vi "trainConGan.vi"(0 "error in (no error)":errorcluster, 1 "ptr_D":i64, 3 "ptr_G":i64, 4 "eta_D":sgl, 5 "eta_G":sgl, 7 "batch_update":u32, 8 "rmsProp":bool=TRUE, 9 "gamma":sgl, 10 "X":sgl[][](array[numeric]), 11 "Y":sgl[][](array[numeric]), 12 "adam":bool=TRUE, 13 "lambda":sgl, 14 "spectral norm discriminator":bool=TRUE, 15 "first Layer":u32, 16 "weight norm Generator":bool=TRUE, 17 "last layer":u32, 18 "train Gen":bool=TRUE, 19 "Gen to sidechannel":bool=TRUE, 27 "handOverLayer":u32) -> (20 "error out":errorcluster, 21 "ptr_D out":i64, 23 "ptr_G out":i64, 24 "Generator output":sgl[][](array[numeric]), 25 "D_REAL_ERR":sgl, 26 "D_FAKE_ERR":sgl)   [LabVIEW 2016, in "CNet.lvlib"]
uses:
  CNet.lvlib
  Users/jg754/Documents/Visual Studio 2015/Projects/CLearn/x64/Release/CLearn.dll
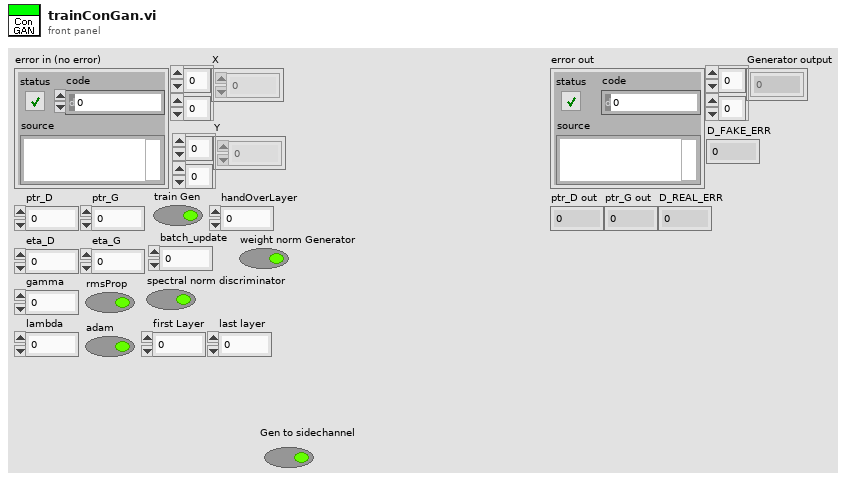
[diagram p1: front panel]
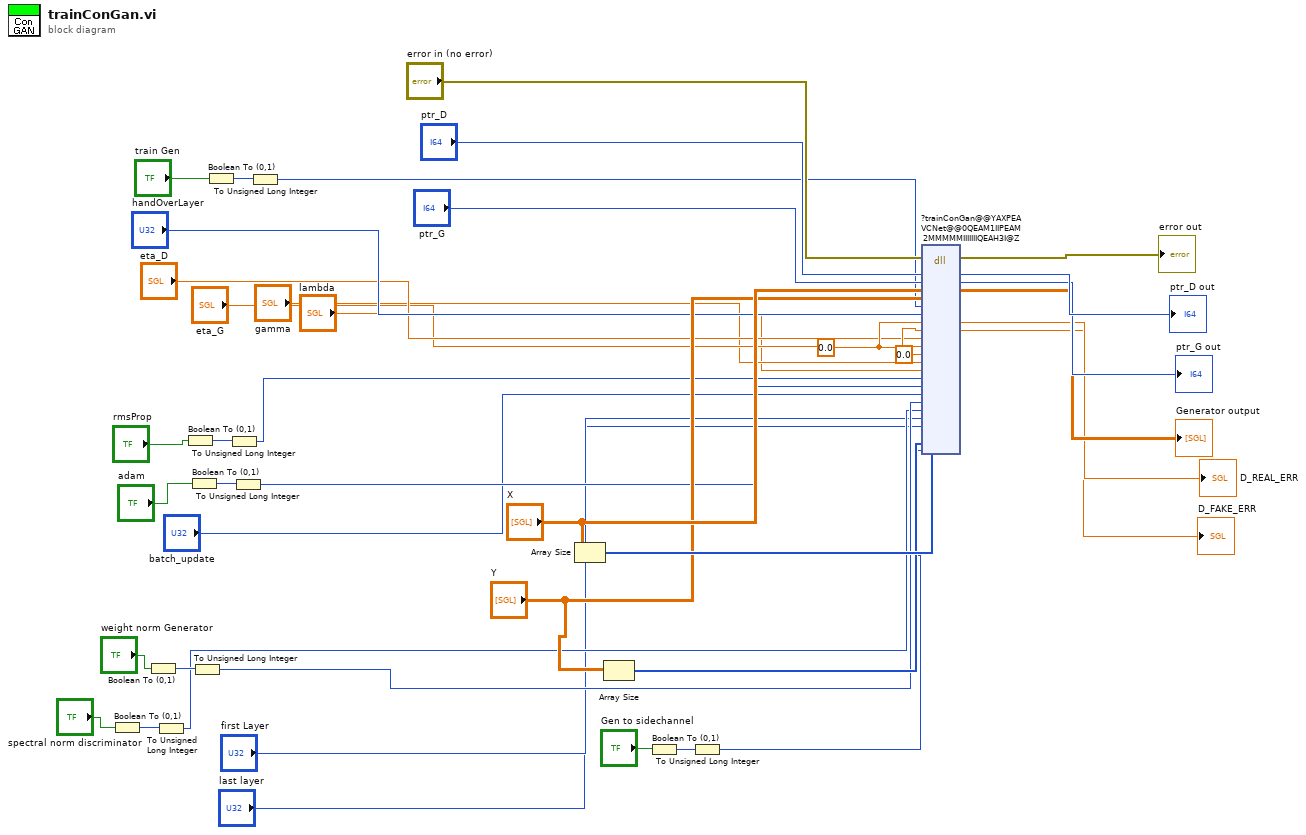
[diagram p0: block diagram]
diagram:
  w26 = sgl 0.0 ("D_REAL_ERR")
  n1 = Boolean To (0,1)(Boolean="spectral norm discriminator") -> (0, 1=w10:i16)
  n2 = Boolean To (0,1)(Boolean="weight norm Generator") -> (0, 1=w13:i16)
  n3 = To Unsigned Long Integer(number=w10) -> (unsigned 32bit integer=w8:u32)
  n4 = Boolean To (0,1)(Boolean="rmsProp") -> (0, 1=w20:i16)
  n5 = Boolean To (0,1)(Boolean="adam") -> (0, 1=w17:i16)
  n6 = To Unsigned Long Integer(number=w13) -> (unsigned 32bit integer=w11:u32)
  n7 = Boolean To (0,1)(Boolean="train Gen") -> (0, 1=w29:i16)
  n8 = To Unsigned Long Integer(number=w20) -> (unsigned 32bit integer=w18:u32)
  n9 = To Unsigned Long Integer(number=w17) -> (unsigned 32bit integer=w15:u32)
  n10 = To Unsigned Long Integer(number=w29) -> (unsigned 32bit integer=w28:u32)
  n11 = Array Size(array="X") -> (size(s)=w34:i32[])
  n12 = Array Size(array="Y") -> (size(s)=w32:i32[])
  n13 = Boolean To (0,1)(Boolean="Gen to sidechannel") -> (0, 1=w2:i16)
  n14 = To Unsigned Long Integer(number=w2) -> (unsigned 32bit integer=w1:u32)
  n15 = dll-call lib="C:/Users/jg754/Documents/Visual Studio 2015/Projects/CLearn/x64/Release/CLearn.dll" fn="?trainConGan@@YAXPEAVCNet@@0QEAM1IIPEAM2MMMMMIIIIIIIQEAH3I@Z"(error in="error in (no error)", "ptr_D"="ptr_D", "ptr_G"="ptr_G", "X"="X", "Y"="Y", "prepGen"=w28, "handOverLayer"="handOverLayer", "D_REAL_ERR"=w26, "D_FAKE_ERR"=w26, "eta_D"="eta_D", "eta_G"="eta_G", "clip"=sgl 0.0, "gamma"="gamma", "lambda"="lambda", "rmsprop"=w18, "adam"=w15, "batch_update"="batch_update", "weight_norm"=w11, "spectral_norm"=w8, "first Layer"="first Layer", "last layer"="last layer", "xFormat"=w34, "yFormat"=w32, "GEN_TO_SIDECHANNEL"=w1) -> (error out=→"error out":errorcluster, "ptr_D"=→"ptr_D out":i64, "ptr_G"=→"ptr_G out":i64, "X"=→"Generator output":sgl[][], "D_REAL_ERR"=→"D_REAL_ERR":sgl, "D_FAKE_ERR"=→"D_FAKE_ERR":sgl)  [unwired: 21 in, 1 out]
